vi "NOYITO-2ChannelRelayControl_LCUS_X2.vi"(6 "RelayControlHexCMD":T1(ring), 8 "error in (no error)":errorcluster, 10 "Baudrate":u32(ring)=9600 items=["4800"=4800, "9600"=9600, "19200"=19200, "38400"=38400, "57600"=57600], 11 "NOYITO-2CH COM":refnum<visa-resource-name>) -> (0 "error out":errorcluster, 1 "RelayResponse":string, 3 "Success":bool)   [LabVIEW 2020, in "NOYITO 2 Channel Relay Driver.lvlib"]
uses:
  <vilib>/Instr/_visa.llb/VISA Configure Serial Port (Instr).vi
  NOYITO 2 Channel Relay Driver.lvlib
panel:
  # "OPEN --> Turns Relay \"ON\"\n\nCLOSED --> Turns Relay \"OFF\""
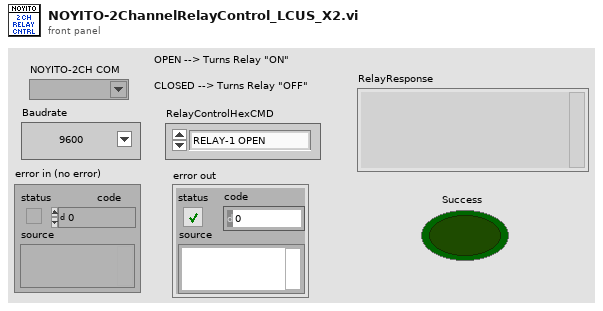
[diagram p1: front panel]
types:
  T1 = enum16{"RELAY-1 OPEN", "RELAY-1 CLOSED", "RELAY-2 OPEN", "RELAY-2 CLOSED", "GET RELAY STATUS"}
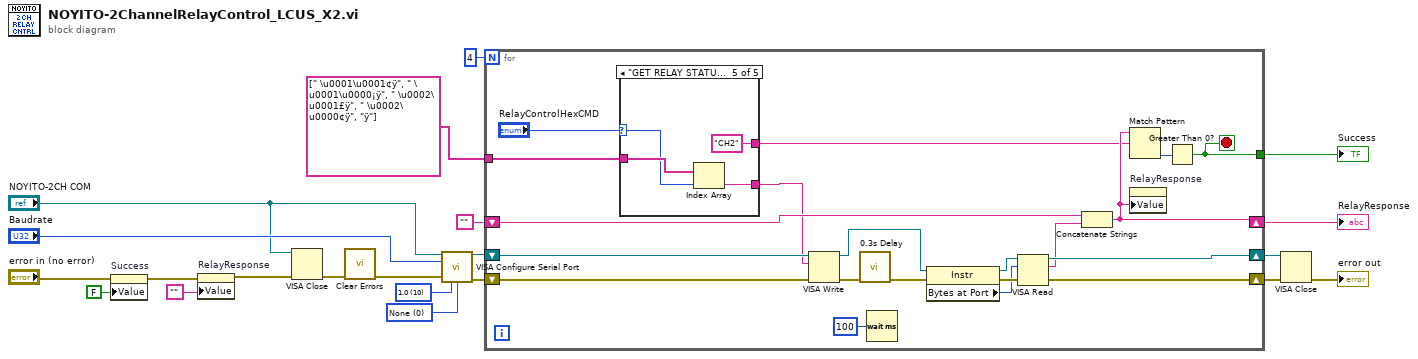
[diagram p0: block diagram]
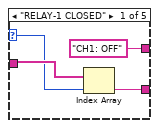
[diagram p2: hidden frame]
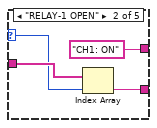
[diagram p3: hidden frame]
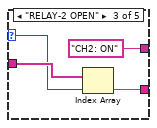
[diagram p4: hidden frame]
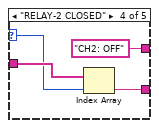
[diagram p5: hidden frame]
diagram:
  w20 = u16 10 items=["1.0"=10, "1.5"=15, "2.0"=20] ("stop bits (10: 1 bit)")
  w21 = u16 0 items=["None", "XON/XOFF", "RTS/CTS", "XON/XOFF & RTS/CTS", "DTR/DSR", "XON/XOFF & DTR/DSR"] ("flow control (0:none)")
  n1 = property on="Success" class="Bool (strict)"(error in="error in (no error)", "Value"=FALSE ("Success")) -> (error out=w3:errorcluster)  [unwired: 1 in, 1 out]
  n2 = property on="RelayResponse" class="Str"(error in=w3, "Value"="") -> (error out=w8:errorcluster)  [unwired: 1 in, 1 out]
  n3 = VISA Close(VISA resource name="NOYITO-2CH COM", error in (no error)=w8) -> (error out=w12:errorcluster)
  n4 = call <vilib>:"Clear Errors.vi"("error in (no error)"=w12) -> ("error out"=w13:errorcluster)  [unwired: 5 in, 1 out]
  n5 = call-poly "VISA Configure Serial Port"("VISA resource name"="NOYITO-2CH COM", "baud rate (9600)"="Baudrate", "error in (no error)"=w13, "stop bits (10: 1 bit)"=w20, "flow control (0:none)"=w21) -> ("VISA resource name out"=w17:refnum<visa-resource-name>, "error out"=w18:errorcluster)  [unwired: 9 in]
  n6 = for {
    N: 4 -> [_]
    shift-right: [w39] -> w16
    shift-left: w18 -> [w41]
    shift-right: [w38] -> w15
    shift-left: w17 -> [w40]
    shift-right: [w25] -> w10
    shift-left: "" -> [w37]
    tunnel: string[] [" \u0001\u0001¢ÿ", " \u0001\u0000¡ÿ", " \u0002\u0001£ÿ", " \u0002\u0000¢ÿ", "ÿ"] -> [w35]
    tunnel: [w22] -> w4
    stop <- w22 stop-if-true
    n7 = case shown="\"GET RELAY STATUS\"" "RelayControlHexCMD" {
      selector: "RelayControlHexCMD" -> [w43 w47 w51 w55 w59]
      tunnel: w35 -> [w44 w48 w52 w56 w60]
      tunnel: [w45 w49 w53 w57 w61] -> w34
      tunnel: ["CH1: OFF" "CH1: ON" "CH2: ON" "CH2: OFF" "CH2"] -> w24
      frame "RELAY-1 CLOSED" {
        n8 = Index Array(array=w44, index=w43) -> (element=w45:string)
      }
      frame "RELAY-1 OPEN" {
        n9 = Index Array(array=w48, index=w47) -> (element=w49:string)
      }
      frame "RELAY-2 OPEN" {
        n10 = Index Array(array=w52, index=w51) -> (element=w53:string)
      }
      frame "RELAY-2 CLOSED" {
        n11 = Index Array(array=w56, index=w55) -> (element=w57:string)
      }
      frame "GET RELAY STATUS" {
        n12 = Index Array(array=w60, index=w59) -> (element=w61:string)
      }
    }
    n13 = VISA Write(VISA resource name=w40, write buffer=w34, error in (no error)=w41) -> (VISA resource name out=w30:refnum<visa-resource-name>, error out=w32:errorcluster)  [unwired: 1 out]
    n14 = call "0.3s Delay"("error in (no error)"=w32) -> ("error out"=w31:errorcluster)  [unwired: 10 in]
    n15 = Wait (ms)(milliseconds to wait=u32 100) -> ()  [unwired: 1 out]
    n16 = property class="Instr"(reference=w30, error in=w31) -> (reference out=w29:refnum<visa-resource-name>, error out=w28:errorcluster, "Bytes at Port"=w27:u32)
    n17 = VISA Read(VISA resource name=w29, byte count=w27, error in (no error)=w28) -> (VISA resource name out=w38:refnum<visa-resource-name>, read buffer=w26:string, error out=w39:errorcluster)  [unwired: 1 out]
    n18 = Concatenate Strings(w37, w26) -> (w25:string)
    n19 = Match Pattern(string=w25, regular expression=w24) -> (offset past match=w23:i32)  [unwired: 1 in, 3 out]
    n20 = property on="RelayResponse" class="Str"("Value"=w25) -> ()  [unwired: 2 in, 2 out]
    n21 = Greater Than 0?(x=w23) -> (x > 0?=w22:bool)
  }
  "RelayResponse" <- w10
  "Success" <- w4
  n22 = VISA Close(VISA resource name=w15, error in (no error)=w16) -> (error out=→"error out":errorcluster)
